vi "LSX Get TVR Out Mode.vi"(0 "lLSID":i32, 1 "plRT":i32, 5 "plXT":i32, 7 "plYT":i32, 9 "plZT":i32, 11 "error in (no error)":errorcluster) -> (3 "plRT out":i32, 4 "function return":i32, 6 "plXT out":i32, 8 "plYT out":i32, 10 "plZT out":i32, 15 "error out":errorcluster)   [LabVIEW 2018, in "Tango.lvlib"]
doc: "TANGOAPI int TANGOCALL LSX_GetTVROutMode (int lLSID, int *plXT, int *plYT, int *plZT, int *plRT);"
uses:
  Tango.lvlib
  SubVIs/Tango_DLL.dll
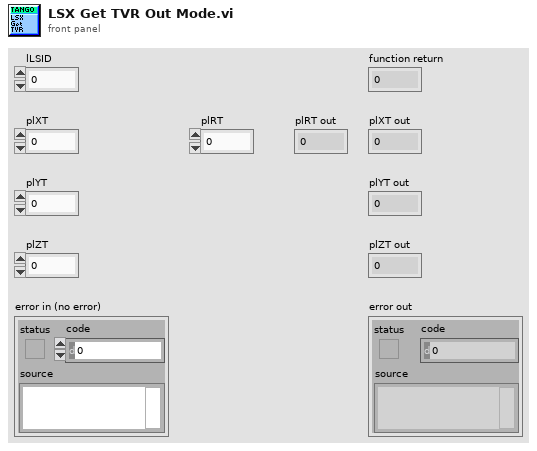
[diagram p1: front panel]
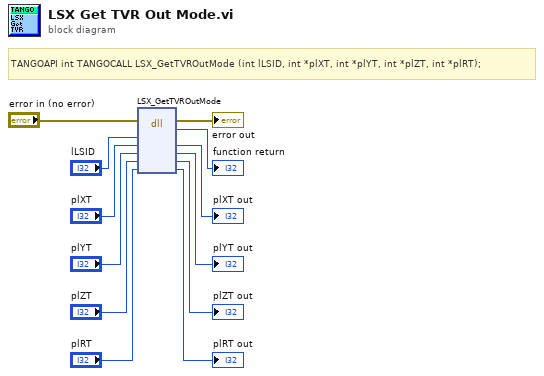
[diagram p0: block diagram]
diagram:
  # "TANGOAPI int TANGOCALL LSX_GetTVROutMode (int lLSID, int *plXT, int *plYT, int *plZT, int *plRT);"
  n1 = dll-call lib="C:/Users/Familie/Documents/LabviewIX81/lib/TANGO Stage/SubVIs/Tango_DLL.*" fn="LSX_GetTVROutMode"(error in="error in (no error)", "lLSID"="lLSID", "plXT"="plXT", "plYT"="plYT", "plZT"="plZT", "plRT"="plRT") -> (error out=→"error out":errorcluster, →"function return":i32, "plXT"=→"plXT out":i32, "plYT"=→"plYT out":i32, "plZT"=→"plZT out":i32, "plRT"=→"plRT out":i32)  [unwired: 3 in, 1 out]
